vi "non_FPGA_VI.vi"() -> ()   [LabVIEW 2020]
uses:
  c5c29772-c0b0-45e0-ac49-cc5077cfdad3.vi
  <vilib>/Array/Sort 2D Array - Pop Stack.vi
  <vilib>/Array/Sort 2D Array - Push Stack.vi
  c5c29772-c0b0-45e0-ac49-cc5077cfdad3.vi/269d4b3b-47f5-49e3-8884-44851e4dd9d5.vi
  c5c29772-c0b0-45e0-ac49-cc5077cfdad3.vi/6d99389c-673d-4efb-bf33-19b32bcf4cf8.vi
  <vilib>/Analysis/NI_AALBase.lvlib
panel:
  out "sorted array":sgl[](graph)
  out "index":i32[](array[numeric])
  out "A Sorted":sgl[](array[numeric])
  out "sorted 2D array":dbl[][](array[numeric])
  out "appended array":dbl[][](array[numeric])
  out "sorted array":dbl[](array[numeric])
  out "uniform white noise":dbl[](array[numeric])
  out "array input":dbl[](graph)
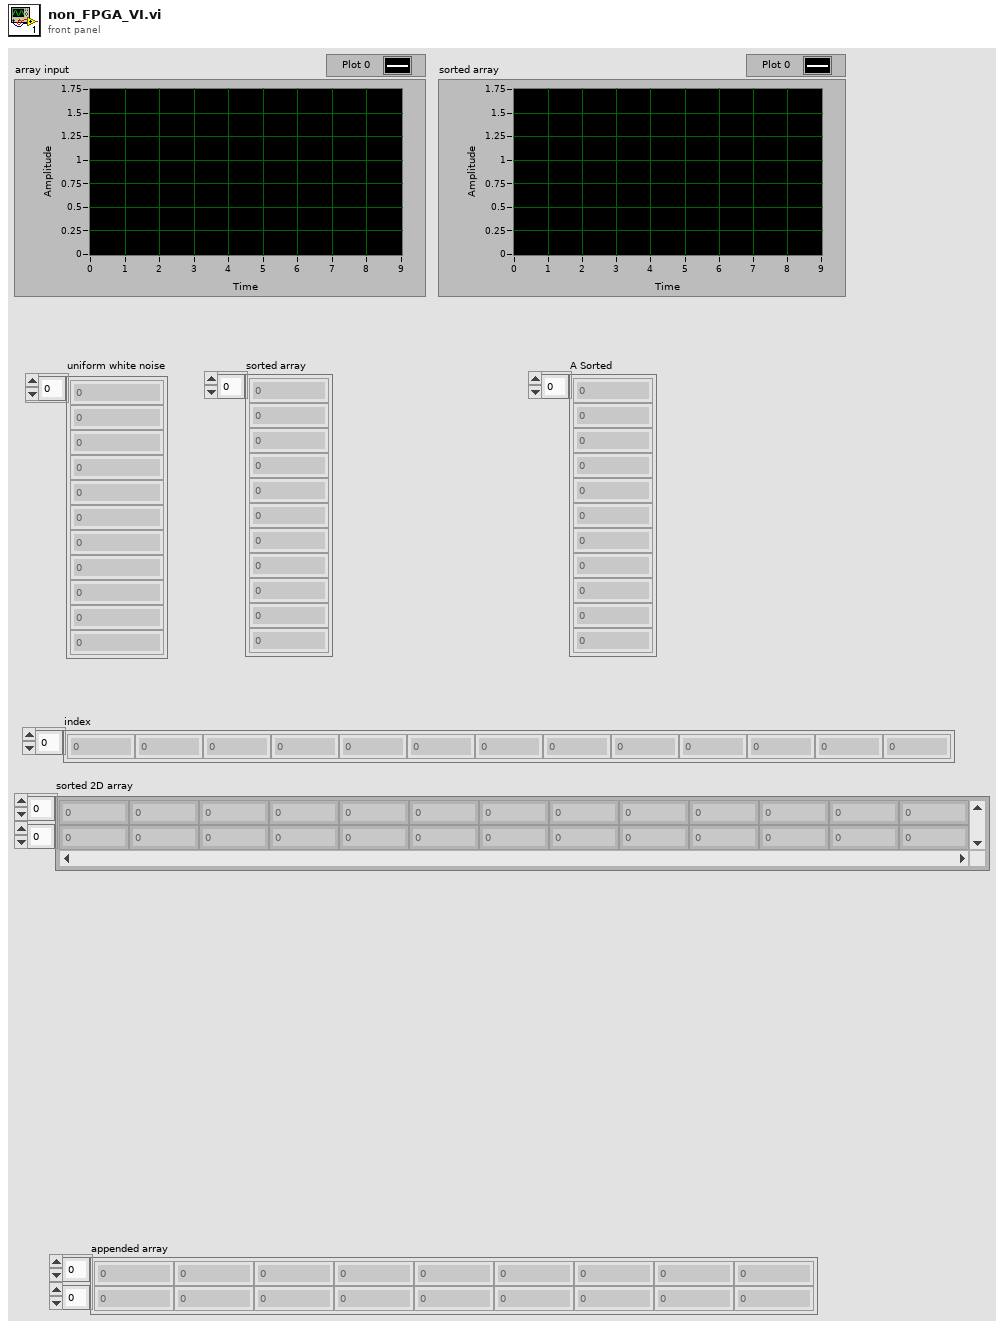
[diagram p1: front panel]
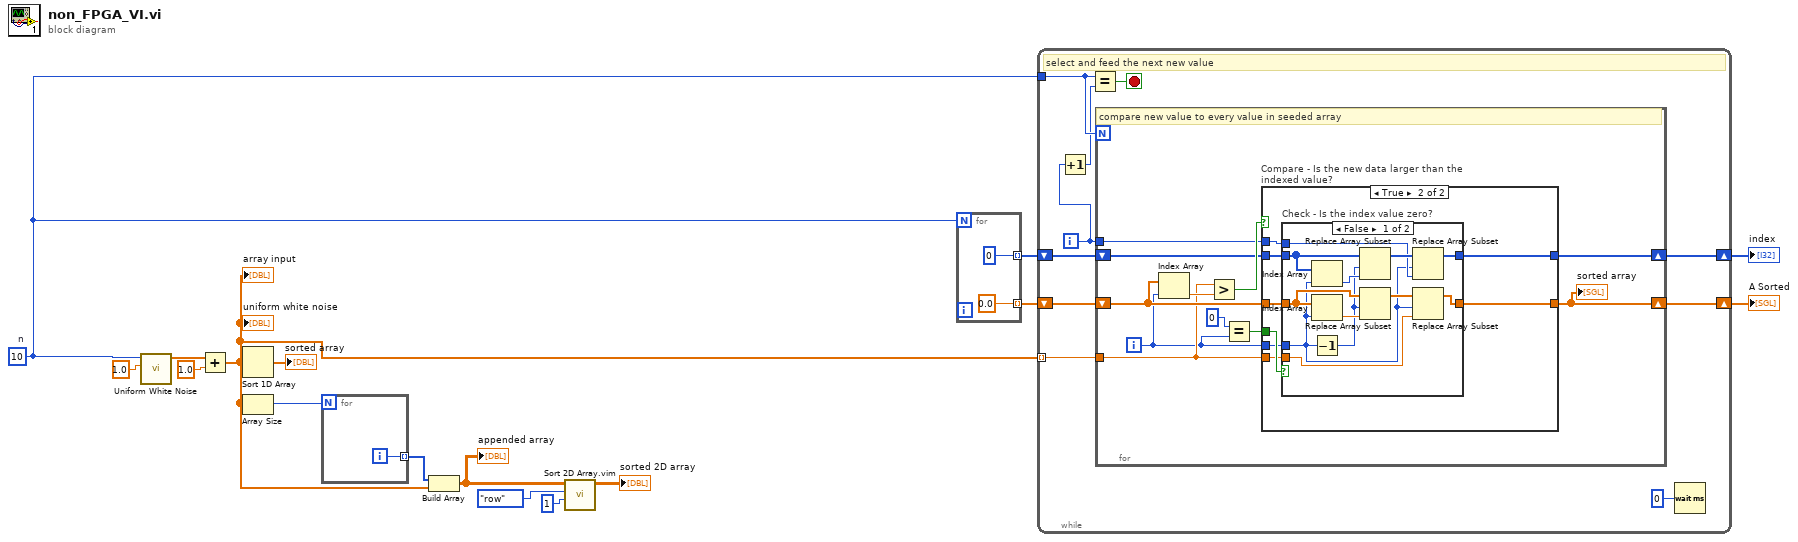
[diagram p0: block diagram]
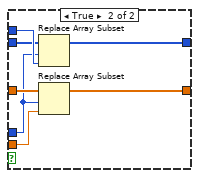
[diagram p3: hidden frame]
diagram:
  w1 = 10  # n
  n1 = call <vilib>:"Uniform White Noise.vi"("amplitude"=1.0, "samples"=w1) -> ("uniform white noise"=w12:dbl[])  [unwired: 8 in, 1 out]
  n2 = Add(x=w12, y=1.0 ("amplitude")) -> (x+y=w3:dbl[])
  "array input" <- w3
  "uniform white noise" <- w3
  n3 = Sort 1D Array(array=w3) -> (sorted array=→"sorted array":dbl[])
  n4 = Array Size(array=w3) -> (size(s)=w13:i32)
  n5 = for {
    N: w13 -> [_]
    tunnel: [w17] -> w11 mode=indexing
    i -> [w17]
  }
  n6 = Build Array(w11, w3) -> (w10:dbl[][])
  "appended array" <- w10
  n7 = call "Sort 2D Array.vim"("index"=1, "dimension to index (column)"=enum16{"column", "row"}."row", "2D array"=w10) -> ("sorted 2D array"=→"sorted 2D array":dbl[][])  [unwired: 7 in, 1 out]
  n8 = for {
    N: w1 -> [_]
    tunnel: [sgl 0.0 ("REAL")] -> w5 mode=indexing
    tunnel: [0 ("INDEX")] -> w6 mode=indexing
  }
  n9 = while {
    shift-right: [w25] -> w2
    shift-left: w5 -> [w29]
    shift-right: [w28] -> w4
    shift-left: w6 -> [w27]
    tunnel: w3 -> [w23] mode=indexing
    tunnel: w1 -> [w22]
    i -> [w21]
    stop <- w26 stop-if-true
    # "select and feed the next new value"
    n10 = Increment(x=w21) -> (x+1=w20:i32)
    n11 = Equal?(x=w22, y=w20) -> (x = y?=w26:bool)
    n12 = for {
      N: w22 -> [_]
      tunnel: w23 -> [w37]
      shift-right: [w36] -> w25
      shift-left: w29 -> [w38]
      tunnel: w21 -> [w34]
      shift-right: [w32] -> w28
      shift-left: w27 -> [w33]
      i -> [w35]
      # "compare new value to every value in seeded array"
      n13 = Index Array(array=w38, index=w35) -> (element=w40:sgl)
      n14 = Greater?(x=w37, y=w40) -> (0:w39:bool)
      n15 = Equal?(x=0, y=w35) -> (x = y?=w30:bool)
      n16 = case "Compare - Is the new data larger than the indexed value?" shown="True" w39 {
        tunnel: w38 -> [w42 w49]
        tunnel: w30 -> [_ w50]
        tunnel: w37 -> [_ w48]
        tunnel: w35 -> [_ w47]
        tunnel: [w42 w46] -> w36
        tunnel: w34 -> [_ w45]
        tunnel: w33 -> [w41 w44]
        tunnel: [w41 w43] -> w32
        frame False {
        }
        frame True {
          n17 = case "Check - Is the index value zero?" shown="False" w50 {
            tunnel: w49 -> [w62 w69]
            tunnel: w48 -> [w59 w68]
            tunnel: w47 -> [w51 w63]
            tunnel: [w58 w67] -> w46
            tunnel: w45 -> [w53 w66]
            tunnel: w44 -> [w55 w65]
            tunnel: [w54 w64] -> w43
            frame False {
              n18 = Index Array(array=w55, index=w51) -> (element=w57:i32)
              n19 = Index Array(array=w62, index=w51) -> (element=w61:sgl)
              n20 = Decrement(x=w51) -> (x-1=w52:i32)
              n21 = Replace Array Subset(array=w55, new element=w57, index=w52) -> (w56:i32[])
              n22 = Replace Array Subset(array=w62, new element=w61, index=w52) -> (w60:sgl[])
              n23 = Replace Array Subset(array=w56, new element=w53, index=w51) -> (w54:i32[])
              n24 = Replace Array Subset(array=w60, new element=w59, index=w51) -> (w58:sgl[])
            }
            frame True {
              n25 = Replace Array Subset(array=w65, new element=w66, index=w63) -> (w64:i32[])
              n26 = Replace Array Subset(array=w69, new element=w68, index=w63) -> (w67:sgl[])
            }
          }
        }
      }
      "sorted array" <- w36
    }
    n27 = Wait (ms)(milliseconds to wait=u32 0) -> ()  [unwired: 1 out]
  }
  "A Sorted" <- w2
  "index" <- w4
